vi "kalman_int_v3.vi"(4 "y_offset":fxp<+/-,16,8>, 5 "x_offset":fxp<+/-,16,8>, 6 "reset":bool, 7 "new_offset":bool, 8 "var_x":fxp<+,16,4>, 9 "var_y":fxp<+,16,4>, 10 "accn_noise":fxp<+,16,16>, 11 "feedback_time (ms)":fxp<+,16,1>) -> (0 "q2_ready":bool, 1 "Q2_update":fxp<+/-,16,8>, 2 "q1_ready":bool, 3 "Q1_update":fxp<+/-,16,8>)   [LabVIEW 2020]
panel:
  out "output valid 44":bool
  out "Pup44":fxp<+,32,16>
  out "output valid 42":bool
  out "Pup42":fxp<+,32,16>
  out "output valid 33":bool
  out "Pup33":fxp<+,32,16>
  out "output valid 31":bool
  out "Pup31":fxp<+,32,16>
  out "output valid 24":bool
  out "Pup24":fxp<+,32,16>
  out "output valid 22":bool
  out "Pup22":fxp<+,32,16>
  out "output valid 13":bool
  out "Pup13":fxp<+,32,16>
  out "output valid 11":bool
  out "Pup11":fxp<+,32,16>
  out "Q2temp_out":fxp<+/-,32,16>
  out "Q1temp_out":fxp<+/-,32,16>
  out "Q4_orig":fxp<+/-,32,16>
  out "Q3_orig":fxp<+/-,32,16>
  out "Q2 orig":fxp<+/-,32,16>
  out "Q1 orig":fxp<+/-,32,16>
  out "q4_ready":bool
  out "Q4_update":fxp<+/-,16,8>
  out "q3_ready":bool
  out "Q3_update":fxp<+/-,16,8>
  out "Q4":fxp<+/-,32,16>
  out "Q3":fxp<+/-,32,16>
  out "Q2":fxp<+/-,32,16>
  out "Q1":fxp<+/-,32,16>
  out "output valid 42":bool
  out "K42":fxp<+,32,16>
  out "output valid 31":bool
  out "K31":fxp<+,32,16>
  out "output valid 22":bool
  out "K22":fxp<+,32,16>
  out "output valid 11":bool
  out "K11":fxp<+,32,16>
  out "new_P24":fxp<+,32,16>
  out "new_P42":fxp<+,32,16>
  out "new_P31":fxp<+,32,16>
  out "new_P13":fxp<+,32,16>
  out "new_P44":fxp<+,32,16>
  out "new_P33":fxp<+,32,16>
  out "new_P22":fxp<+,32,16>
  out "new_P11":fxp<+,32,16>
  out "E31":fxp<+,32,16>
  out "E33":fxp<+,32,16>
  out "E11":fxp<+,32,16>
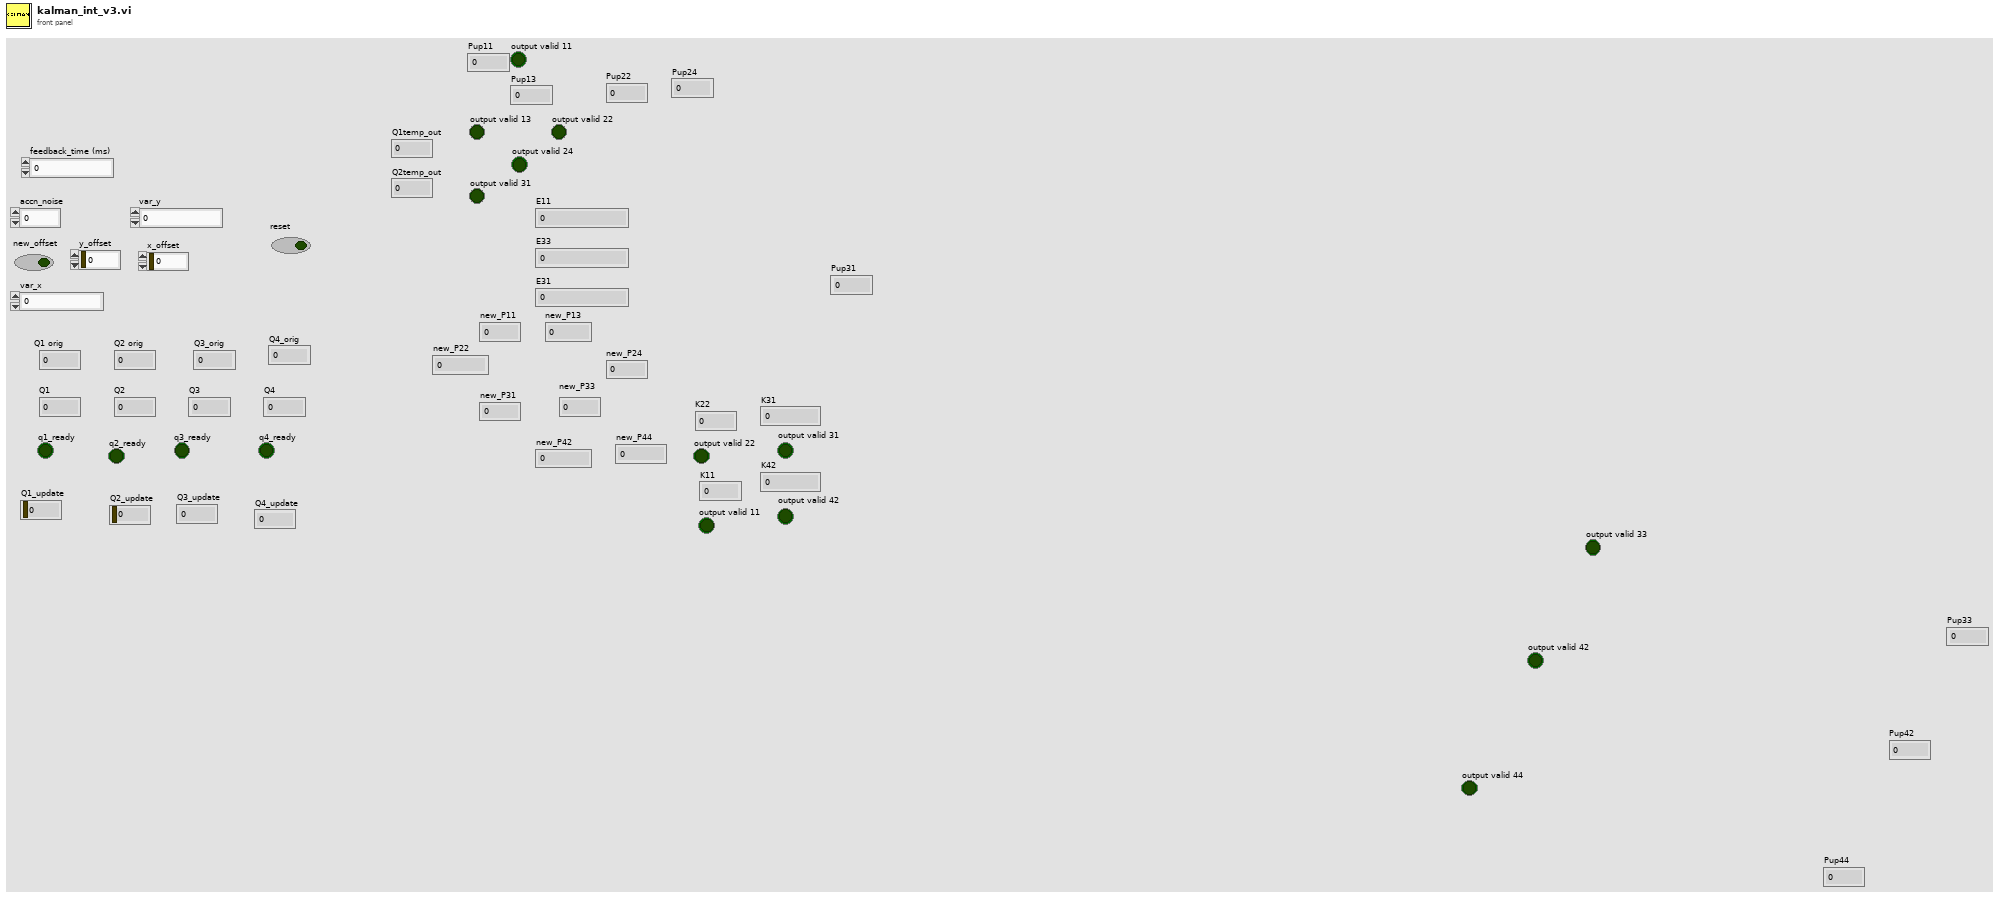
[diagram p1: front panel]
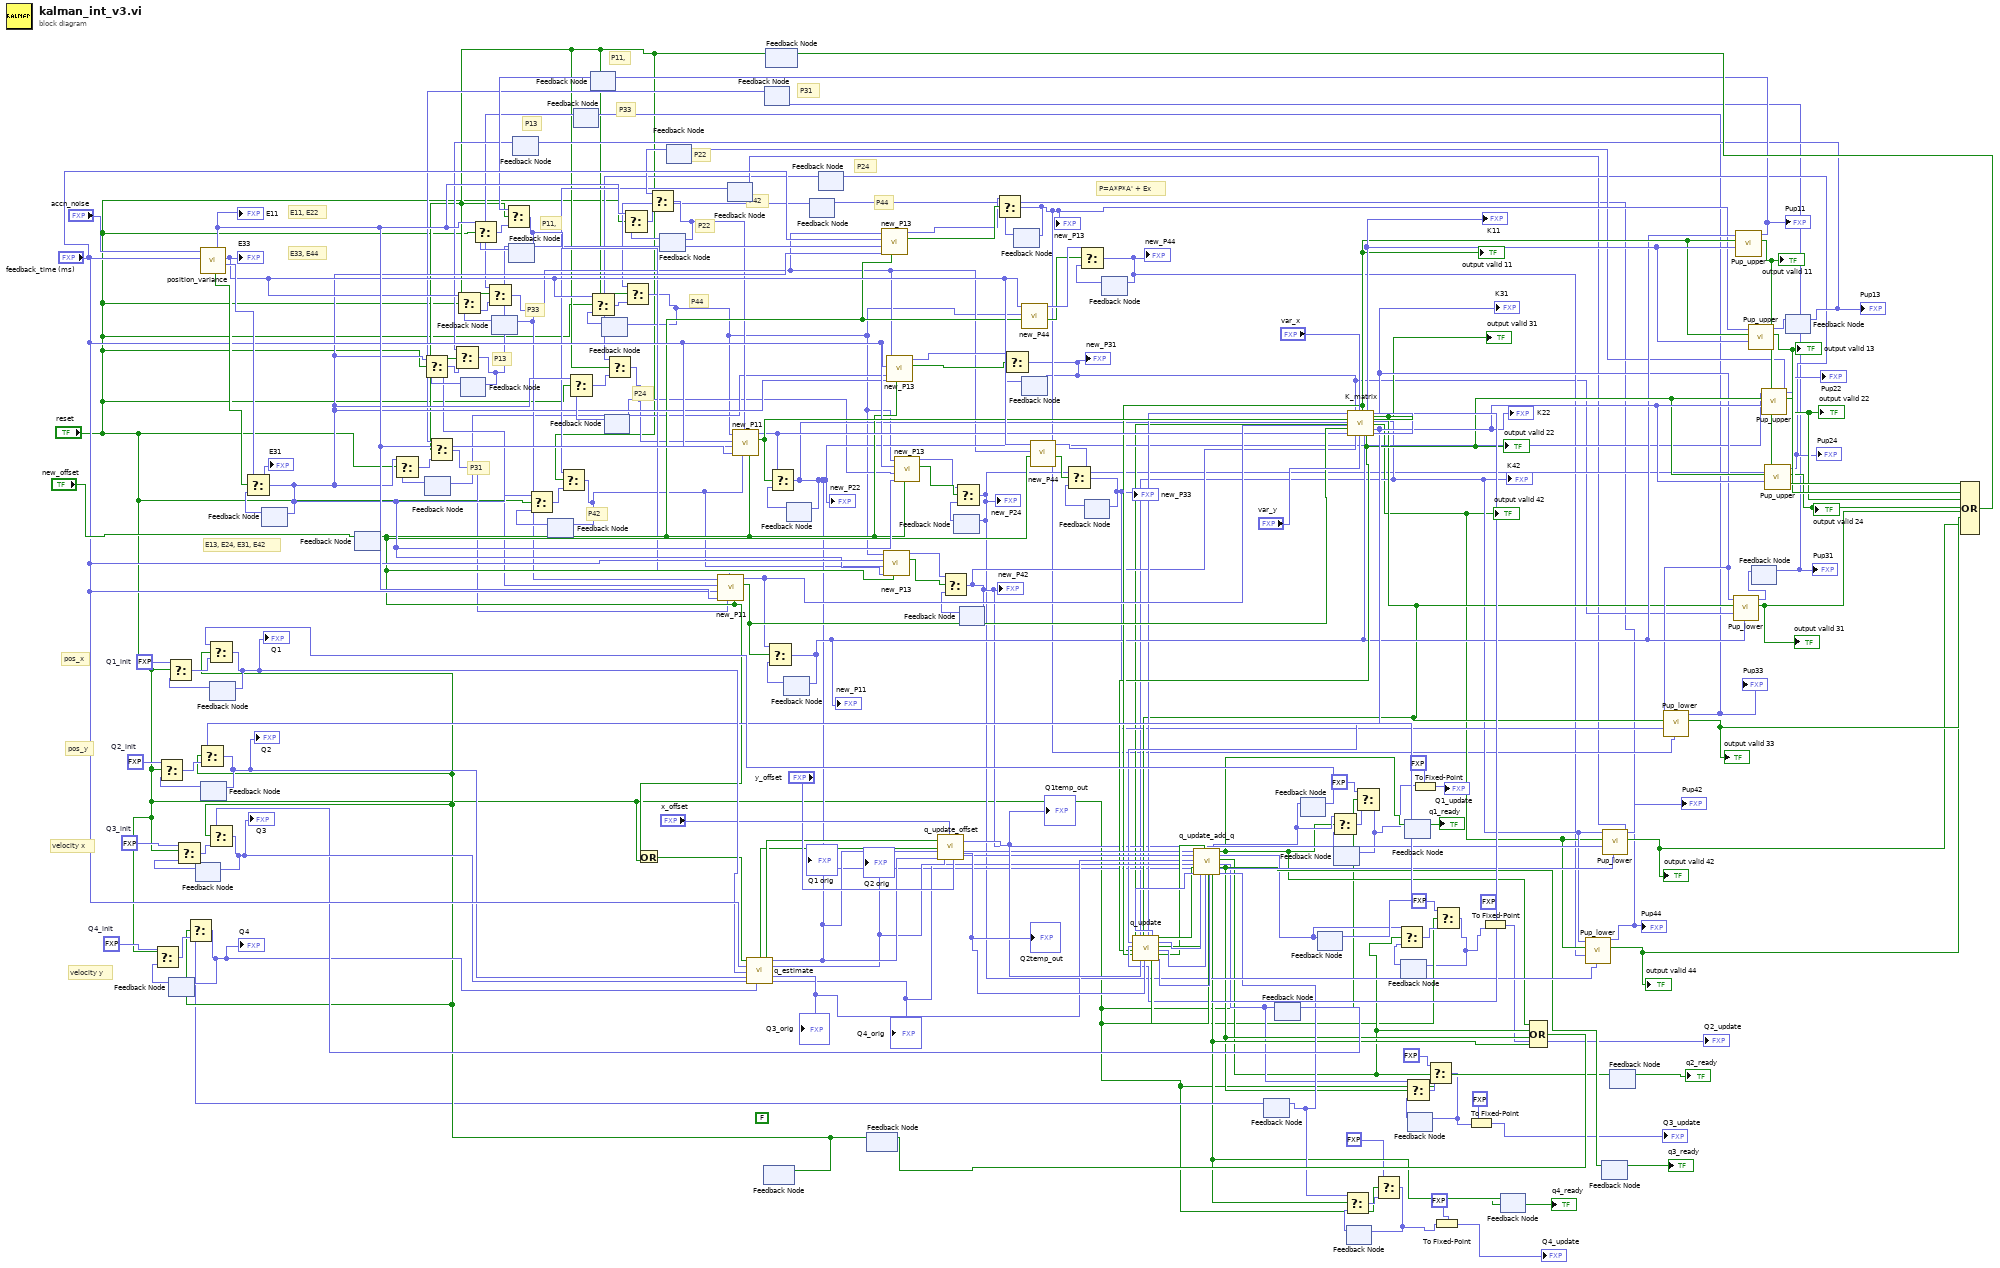
[diagram p0: block diagram]
diagram:
  (unwired) FALSE
  w135 = fxp<+/-,32,16> 0.0  # Q4_init
  w137 = fxp<+/-,32,16> 0.0  # Q3_init
  w139 = fxp<+/-,32,16> 0.0  # Q2_init
  w141 = fxp<+/-,32,16> 0.0  # Q1_init
  # "P22"
  # "P44"
  # "P42"
  # "P33"
  # "P31"
  # "P24"
  # "P13"
  # "P11,"
  # "velocity y"
  # "velocity x"
  # "pos_y"
  # "pos_x"
  # "P=A*P*A' + Ex"
  # "P42"
  # "P31"
  # "P24"
  # "P44"
  # "P22"
  # "P13"
  # "P33"
  # "P11,"
  # "E13, E24, E31, E42"
  # "E33, E44"
  # "E11, E22"
  n1 = feedback #1() -> (w134:fxp<+/-,32,16>)  [unwired: 1 in]
  n2 = Select(t=w135, s="reset", f=w134) -> (s? t:f=w123:fxp<+/-,32,16>)
  n3 = feedback #2() -> (w136:fxp<+/-,32,16>)  [unwired: 1 in]
  n4 = Select(t=w137, s="reset", f=w136) -> (s? t:f=w126:fxp<+/-,32,16>)
  n5 = call "position_variance.vi"("feedback_time (ms)"="feedback_time (ms)", "accn_noise"="accn_noise") -> ("E31"=w170:fxp<+,32,16>, "E33"=w168:fxp<+,32,16>, "E11"=w173:fxp<+,32,16>, "output valid"=w172:bool)  [unwired: 6 in]
  "E11" <- w173
  "E33" <- w168
  n6 = feedback #3() -> (w138:fxp<+/-,32,16>)  [unwired: 1 in]
  n7 = Select(t=w139, s="reset", f=w138) -> (s? t:f=w129:fxp<+/-,32,16>)
  n8 = feedback #4() -> (w140:fxp<+/-,32,16>)  [unwired: 1 in]
  n9 = Select(t=w141, s="reset", f=w140) -> (s? t:f=w132:fxp<+/-,32,16>)
  n10 = feedback #5() -> (w171:fxp<+,32,16>)  [unwired: 1 in]
  n11 = Select(t=w170, s=w172, f=w171) -> (s? t:f=w103:fxp<+,32,16>)
  "E31" <- w103
  n12 = feedback-in #5(w103) -> ()
  n13 = feedback #6() -> (w100:bool)  [unwired: 1 in]
  n14 = feedback-in #6("new_offset") -> ()
  n15 = feedback #7() -> (w175:fxp<+,32,16>)  [unwired: 1 in]
  n16 = Select(t=w103, s="reset", f=w175) -> (s? t:f=w48:fxp<+,32,16>)
  n17 = feedback #8() -> (w179:fxp<+,32,16>)  [unwired: 1 in]
  n18 = Select(t=w103, s="reset", f=w179) -> (s? t:f=w60:fxp<+,32,16>)
  n19 = feedback #9() -> (w180:fxp<+,32,16>)  [unwired: 1 in]
  n20 = Select(t=w168, s="reset", f=w180) -> (s? t:f=w57:fxp<+,32,16>)
  n21 = feedback #10() -> (w181:fxp<+,32,16>)  [unwired: 1 in]
  n22 = Select(t=w173, s="reset", f=w181) -> (s? t:f=w63:fxp<+,32,16>)
  n23 = feedback #11() -> (w58:fxp<+,32,16>)  [unwired: 1 in]
  n24 = feedback #12() -> (w174:fxp<+,32,16>)  [unwired: 1 in]
  n25 = Select(t=w103, s="reset", f=w174) -> (s? t:f=w51:fxp<+,32,16>)
  n26 = feedback #13() -> (w55:fxp<+,32,16>)  [unwired: 1 in]
  n27 = feedback #14() -> (w61:fxp<+,32,16>)  [unwired: 1 in]
  n28 = feedback #15() -> (w177:fxp<+,32,16>)  [unwired: 1 in]
  n29 = Select(t=w168, s="reset", f=w177) -> (s? t:f=w42:fxp<+,32,16>)
  n30 = feedback #16() -> (w176:fxp<+,32,16>)  [unwired: 1 in]
  n31 = Select(t=w103, s="reset", f=w176) -> (s? t:f=w45:fxp<+,32,16>)
  n32 = Or(x=w100, y="reset") -> (x .or. y?=w99:bool)
  n33 = feedback #17() -> (w178:fxp<+,32,16>)  [unwired: 1 in]
  n34 = Select(t=w173, s="reset", f=w178) -> (s? t:f=w54:fxp<+,32,16>)
  n35 = feedback #18() -> (w52:fxp<+,32,16>)  [unwired: 1 in]
  n36 = feedback #19() -> (w49:fxp<+,32,16>)  [unwired: 1 in]
  n37 = feedback #20() -> ()  [unwired: 2 in]
  n38 = feedback #21() -> (w46:fxp<+,32,16>)  [unwired: 1 in]
  n39 = feedback #22() -> (w40:bool)  [unwired: 1 in]
  n40 = Select(t=w46, s=w40, f=w48) -> (s? t:f=w47:fxp<+,32,16>)
  n41 = feedback-in #7(w47) -> ()
  n42 = Select(t=w58, s=w40, f=w60) -> (s? t:f=w59:fxp<+,32,16>)
  n43 = feedback-in #8(w59) -> ()
  n44 = Select(t=w55, s=w40, f=w57) -> (s? t:f=w56:fxp<+,32,16>)
  n45 = feedback-in #9(w56) -> ()
  n46 = Select(t=w61, s=w40, f=w63) -> (s? t:f=w62:fxp<+,32,16>)
  n47 = feedback-in #10(w62) -> ()
  n48 = Select(t=w49, s=w40, f=w51) -> (s? t:f=w50:fxp<+,32,16>)
  n49 = feedback-in #12(w50) -> ()
  n50 = Select(t=w52, s=w40, f=w54) -> (s? t:f=w53:fxp<+,32,16>)
  n51 = feedback-in #17(w53) -> ()
  n52 = call "new_P11.vi"("Boolean"=w100, "P31"=w47, "P11"=w62, "E11"=w173, "feedback_time (ms)"="feedback_time (ms)", "P13"=w60, "P33"=w56) -> ("output valid"=w156:bool, "P11+dt*P31 + dt*(P13+dt*P33) + E1"=w155:fxp<+,32,16>)  [unwired: 3 in]
  n53 = feedback #23() -> (w154:fxp<+,32,16>)  [unwired: 1 in]
  n54 = Select(t=w155, s=w156, f=w154) -> (s? t:f=w94:fxp<+,32,16>)
  "new_P11" <- w94
  n55 = feedback-in #23(w94) -> ()
  n56 = feedback #24() -> (w151:fxp<+,32,16>)  [unwired: 1 in]
  n57 = feedback #25() -> (w39:fxp<+,32,16>)  [unwired: 1 in]
  n58 = Select(t=w39, s=w40, f=w42) -> (s? t:f=w41:fxp<+,32,16>)
  n59 = feedback-in #15(w41) -> ()
  n60 = feedback #26() -> (w43:fxp<+,32,16>)  [unwired: 1 in]
  n61 = Select(t=w43, s=w40, f=w45) -> (s? t:f=w44:fxp<+,32,16>)
  n62 = feedback-in #16(w44) -> ()
  n63 = call "new_P11.vi"("Boolean"=w100, "P31"=w50, "P11"=w53, "E11"=w173, "feedback_time (ms)"="feedback_time (ms)", "P13"=w44, "P33"=w41) -> ("output valid"=w153:bool, "P11+dt*P31 + dt*(P13+dt*P33) + E1"=w152:fxp<+,32,16>)  [unwired: 3 in]
  n64 = Select(t=w152, s=w153, f=w151) -> (s? t:f=w89:fxp<+,32,16>)
  "new_P22" <- w89
  n65 = feedback-in #24(w89) -> ()
  n66 = feedback #27() -> (w101:bool)  [unwired: 1 in]
  n67 = feedback-in #20(w101) -> ()
  n68 = call "new_P13.vi"("Boolean"=w100, "E13"=w103, "P13"=w59, "feedback_time (ms)"="feedback_time (ms)", "P33"=w56) -> ("output valid"=w165:bool, "P13 + dt*P33 + E13"=w164:fxp<+,32,16>)  [unwired: 5 in]
  n69 = call "new_P13.vi"("Boolean"=w100, "E13"=w103, "P13"=w50, "feedback_time (ms)"="feedback_time (ms)", "P33"=w41) -> ("output valid"=w150:bool, "P13 + dt*P33 + E13"=w149:fxp<+,32,16>)  [unwired: 5 in]
  n70 = call "new_P13.vi"("Boolean"=w100, "E13"=w103, "P13"=w47, "feedback_time (ms)"="feedback_time (ms)", "P33"=w56) -> ("output valid"=w159:bool, "P13 + dt*P33 + E13"=w158:fxp<+,32,16>)  [unwired: 5 in]
  n71 = call "new_P13.vi"("Boolean"=w100, "E13"=w103, "P13"=w44, "feedback_time (ms)"="feedback_time (ms)", "P33"=w41) -> ("output valid"=w147:bool, "P13 + dt*P33 + E13"=w146:fxp<+,32,16>)  [unwired: 5 in]
  n72 = feedback #28() -> (w145:fxp<+,32,16>)  [unwired: 1 in]
  n73 = Select(t=w146, s=w147, f=w145) -> (s? t:f=w86:fxp<+,32,16>)
  "new_P24" <- w86
  n74 = feedback-in #28(w86) -> ()
  n75 = feedback #29() -> (w148:fxp<+,32,16>)  [unwired: 1 in]
  n76 = Select(t=w149, s=w150, f=w148) -> (s? t:f=w90:fxp<+,32,16>)
  "new_P42" <- w90
  n77 = feedback-in #29(w90) -> ()
  n78 = feedback #30() -> (w163:fxp<+,32,16>)  [unwired: 1 in]
  n79 = Select(t=w164, s=w165, f=w163) -> (s? t:f=w74:fxp<+,32,16>)
  "new_P13" <- w74
  n80 = feedback-in #30(w74) -> ()
  n81 = call "new_P44.vi"("new_offset"=w100, "P44"=w41, "E44"=w168) -> ("output valid"=w161:bool, "new_P44"=w162:fxp<+,32,16>)  [unwired: 7 in]
  n82 = feedback #31() -> (w157:fxp<+,32,16>)  [unwired: 1 in]
  n83 = Select(t=w158, s=w159, f=w157) -> (s? t:f=w72:fxp<+,32,16>)
  "new_P31" <- w72
  n84 = feedback-in #31(w72) -> ()
  n85 = call "new_P44.vi"("new_offset"=w100, "P44"=w56, "E44"=w168) -> ("output valid"=w144:bool, "new_P44"=w143:fxp<+,32,16>)  [unwired: 7 in]
  n86 = feedback #32() -> (w142:fxp<+,32,16>)  [unwired: 1 in]
  n87 = Select(t=w143, s=w144, f=w142) -> (s? t:f=w91:fxp<+,32,16>)
  "new_P33" <- w91
  n88 = feedback-in #32(w91) -> ()
  n89 = feedback #33() -> (w160:fxp<+,32,16>)  [unwired: 1 in]
  n90 = Select(t=w162, s=w161, f=w160) -> (s? t:f=w73:fxp<+,32,16>)
  "new_P44" <- w73
  n91 = feedback-in #33(w73) -> ()
  n92 = feedback #34() -> (w38:fxp<+/-,32,16>)  [unwired: 1 in]
  n93 = Select(t=w38, s=w101, f=w123) -> (s? t:f=w122:fxp<+/-,32,16>)
  "Q4" <- w122
  n94 = feedback-in #1(w122) -> ()
  n95 = feedback #35() -> (w124:fxp<+/-,32,16>)  [unwired: 1 in]
  n96 = Select(t=w124, s=w101, f=w126) -> (s? t:f=w125:fxp<+/-,32,16>)
  "Q3" <- w125
  n97 = feedback-in #2(w125) -> ()
  n98 = feedback #36() -> (w130:fxp<+/-,32,16>)  [unwired: 1 in]
  n99 = Select(t=w130, s=w101, f=w132) -> (s? t:f=w131:fxp<+/-,32,16>)
  "Q1" <- w131
  n100 = feedback-in #4(w131) -> ()
  n101 = feedback #37() -> (w127:fxp<+/-,32,16>)  [unwired: 1 in]
  n102 = Select(t=w127, s=w101, f=w129) -> (s? t:f=w128:fxp<+/-,32,16>)
  "Q2" <- w128
  n103 = feedback-in #3(w128) -> ()
  n104 = call "q_estimate.vi"("new_offset"=w99, "feedback_time (ms)"="feedback_time (ms)", "Q1_init"=w131, "Q2_init"=w128, "Q3_init in"=w125, "Q4_init in"=w122) -> ("Q1 temp"=w107:fxp<+/-,32,16>, "Q2 temp"=w106:fxp<+/-,32,16>, "Q3_temp"=w105:fxp<+/-,32,16>, "q1_valid"=w118:bool, "Q2_valid"=w119:bool, "Q4_temp"=w104:fxp<+/-,32,16>)  [unwired: 4 in]
  "Q1 orig" <- w107
  "Q2 orig" <- w106
  "Q3_orig" <- w105
  "Q4_orig" <- w104
  n105 = call "q_update_offset.vi"("Q2 valid"=w119, "Q1 valid"=w118, "Q1_temp"=w107, "Q2_temp"=w106, "x_offset"="x_offset", "y_offset"="y_offset") -> ("Q1temp_out"=w116:fxp<+/-,32,16>, "Q2temp_out"=w117:fxp<+/-,32,16>)  [unwired: 10 in, 2 out]
  "Q1temp_out" <- w116
  "Q2temp_out" <- w117
  n106 = feedback #38() -> (w27:fxp<+/-,32,16>)  [unwired: 1 in]
  n107 = feedback #39() -> (w35:fxp<+/-,32,16>)  [unwired: 1 in]
  n108 = call "K_matrix.vi"("new_P22"=w152, "output valid"=w153, "P22_new"=w89, "new_P11"=w155, "output valid 2"=w156, "P31_new"=w72, "P42_new"=w90, "var_x"="var_x", "var_y"="var_y", "P11_new"=w94) -> ("output valid 11"=w97:bool, "K11"=w98:fxp<+,32,16>, "output valid 22"=w95:bool, "K31"=w93:fxp<+,32,16>, "output valid 31"=w92:bool, "K42"=w88:fxp<+,32,16>, "output valid 42"=w87:bool, "K22"=w96:fxp<+,32,16>)  [unwired: 2 in]
  "K11" <- w98
  "output valid 11" <- w97
  "K22" <- w96
  "output valid 22" <- w95
  "K31" <- w93
  "output valid 31" <- w92
  "K42" <- w88
  "output valid 42" <- w87
  n109 = call "q_update.vi"("output valid 42"=w87, "K22"=w96, "K11"=w98, "output valid 22"=w95, "output valid 11"=w97, "K42"=w88, "Q1_temp off"=w116, "output valid 31"=w92, "Q2_temp off"=w117, "K31"=w93) -> ("Q1_temp"=w115:fxp<+/-,32,16>, "q4_ready"=w108:bool, "q1_ready"=w114:bool, "Q2_temp"=w113:fxp<+/-,32,16>, "q2_ready"=w112:bool, "Q3_temp"=w111:fxp<+/-,32,16>, "q3_ready"=w110:bool, "Q4_update"=w109:fxp<+/-,32,16>)  [unwired: 2 in]
  n110 = call "q_update_add_q.vi"("Q1_orig"=w107, "Q2_orig"=w106, "Q3_orig"=w105, "Q4_orig"=w104, "q1_valid"=w114, "Q1_temp"=w115, "q2_valid"=w112, "Q2_temp"=w113, "q3_valid"=w110, "Q3_temp"=w111, "q4_valid"=w108, "Q4_temp"=w109) -> ("Q1_update"=w28:fxp<+/-,32,16>, "q4_ready"=w36:bool, "q1_ready"=w26:bool, "Q2_update"=w30:fxp<+/-,32,16>, "q2_ready"=w31:bool, "Q3_update"=w33:fxp<+/-,32,16>, "q3_ready"=w34:bool, "Q4_update"=w37:fxp<+/-,32,16>)
  n111 = feedback-in #34(w37) -> ()
  n112 = feedback-in #35(w33) -> ()
  n113 = feedback-in #36(w28) -> ()
  n114 = feedback-in #37(w30) -> ()
  n115 = Select(t=w28, s=w26, f=w27) -> (s? t:f=w18:fxp<+/-,32,16>)
  n116 = Select(t=w37, s=w36, f=w35) -> (s? t:f=w25:fxp<+/-,32,16>)
  n117 = Select(t=fxp<+/-,32,16> 0.0, s="reset", f=w18) -> (s? t:f=w15:fxp<+/-,32,16>)
  n118 = feedback-in #38(w15) -> ()
  n119 = Select(t=fxp<+/-,32,16> 0.0, s="reset", f=w25) -> (s? t:f=w7:fxp<+/-,32,16>)
  n120 = feedback-in #39(w7) -> ()
  n121 = feedback #40() -> (w29:fxp<+/-,32,16>)  [unwired: 1 in]
  n122 = Select(t=w30, s=w31, f=w29) -> (s? t:f=w20:fxp<+/-,32,16>)
  n123 = feedback #41() -> (→"q1_ready":bool)  [unwired: 1 in]
  n124 = feedback-in #41(w26) -> ()
  n125 = feedback #42() -> (w32:fxp<+/-,32,16>)  [unwired: 1 in]
  n126 = Select(t=w33, s=w34, f=w32) -> (s? t:f=w22:fxp<+/-,32,16>)
  n127 = To Fixed-Point(fixed-point type=fxp<+/-,16,8> 0.0, number=w15) -> (fixed-point=→"Q1_update":fxp<+/-,16,8>)
  n128 = Select(t=fxp<+/-,32,16> 0.0, s="reset", f=w22) -> (s? t:f=w9:fxp<+/-,32,16>)
  n129 = feedback-in #42(w9) -> ()
  n130 = To Fixed-Point(fixed-point type=fxp<+/-,16,8> 0.0, number=w7) -> (fixed-point=→"Q4_update":fxp<+/-,16,8>)
  n131 = Select(t=fxp<+/-,32,16> 0.0, s="reset", f=w20) -> (s? t:f=w12:fxp<+/-,32,16>)
  n132 = feedback-in #40(w12) -> ()
  n133 = To Fixed-Point(fixed-point type=fxp<+/-,16,8> 0.0, number=w9) -> (fixed-point=→"Q3_update":fxp<+/-,16,8>)
  n134 = To Fixed-Point(fixed-point type=fxp<+/-,16,8> 0.0, number=w12) -> (fixed-point=→"Q2_update":fxp<+/-,16,8>)
  n135 = feedback #43() -> (→"q4_ready":bool)  [unwired: 1 in]
  n136 = feedback-in #43(w36) -> ()
  n137 = Compound Arithmetic op=OR(w26, w31, w34, w36) -> (w102:bool)
  n138 = feedback-in #27(w102) -> ()
  n139 = call "Pup_lower.vi"("P11+dt*P31 + dt*(P13+dt*P33) + E1"=w86, "P13 + dt*P33 + E13"=w73, "output valid 32"=w87, "K31"=w88) -> ("output valid 31"=w78:bool, "Pup31"=w64:fxp<+,32,16>)  [unwired: 6 in]
  "Pup44" <- w64
  "output valid 44" <- w78
  n140 = feedback-in #25(w64) -> ()
  n141 = feedback #44() -> (→"q3_ready":bool)  [unwired: 1 in]
  n142 = feedback-in #44(w34) -> ()
  n143 = call "Pup_lower.vi"("P11+dt*P31 + dt*(P13+dt*P33) + E1"=w89, "P13 + dt*P33 + E13"=w90, "output valid 32"=w87, "K31"=w88) -> ("output valid 31"=w79:bool, "Pup31"=w65:fxp<+,32,16>)  [unwired: 6 in]
  "Pup42" <- w65
  "output valid 42" <- w79
  n144 = feedback-in #19(w65) -> ()
  n145 = feedback #45() -> (→"q2_ready":bool)  [unwired: 1 in]
  n146 = feedback-in #45(w31) -> ()
  n147 = call "Pup_lower.vi"("P11+dt*P31 + dt*(P13+dt*P33) + E1"=w74, "P13 + dt*P33 + E13"=w91, "output valid 32"=w92, "K31"=w93) -> ("output valid 31"=w80:bool, "Pup31"=w66:fxp<+,32,16>)  [unwired: 6 in]
  "Pup33" <- w66
  "output valid 33" <- w80
  n148 = feedback-in #13(w66) -> ()
  n149 = call "Pup_lower.vi"("P11+dt*P31 + dt*(P13+dt*P33) + E1"=w94, "P13 + dt*P33 + E13"=w72, "output valid 32"=w92, "K31"=w93) -> ("output valid 31"=w81:bool, "Pup31"=w75:fxp<+,32,16>)  [unwired: 6 in]
  "output valid 31" <- w81
  n150 = call "Pup_upper.vi"("K11"=w98, "output valid 12"=w97, "E11"=w94) -> ("output valid 11"=w85:bool, "Pup11"=w71:fxp<+,32,16>)  [unwired: 7 in]
  "Pup11" <- w71
  "output valid 11" <- w85
  n151 = feedback-in #14(w71) -> ()
  n152 = call "Pup_upper.vi"("K11"=w98, "output valid 12"=w97, "E11"=w74) -> ("output valid 11"=w84:bool, "Pup11"=w76:fxp<+,32,16>)  [unwired: 7 in]
  "output valid 13" <- w84
  n153 = feedback #46() -> (w67:fxp<+,32,16>)  [unwired: 1 in]
  "Pup31" <- w67
  n154 = feedback-in #21(w67) -> ()
  n155 = feedback-in #46(w75) -> ()
  n156 = call "Pup_upper.vi"("K11"=w96, "output valid 12"=w95, "E11"=w89) -> ("output valid 11"=w83:bool, "Pup11"=w69:fxp<+,32,16>)  [unwired: 7 in]
  "Pup22" <- w69
  "output valid 22" <- w83
  n157 = feedback-in #18(w69) -> ()
  n158 = call "Pup_upper.vi"("K11"=w96, "output valid 12"=w95, "E11"=w86) -> ("output valid 11"=w82:bool, "Pup11"=w68:fxp<+,32,16>)  [unwired: 7 in]
  "Pup24" <- w68
  "output valid 24" <- w82
  n159 = feedback-in #26(w68) -> ()
  n160 = feedback #47() -> (w70:fxp<+,32,16>)  [unwired: 1 in]
  "Pup13" <- w70
  n161 = feedback-in #11(w70) -> ()
  n162 = feedback-in #47(w76) -> ()
  n163 = Compound Arithmetic op=OR(w85, w84, w83, w82, w81, w80, w79, w78) -> (w77:bool)
  n164 = feedback-in #22(w77) -> ()
